vi "Data_analyzer_tester.vi"() -> ()   [LabVIEW 2021]
uses:
  <vilib>/DAQmx/create/channels.llb/DAQmx Create Channel (AI-Voltage-Basic).vi
  <vilib>/DAQmx/configure/timing.llb/DAQmx Timing (Sample Clock).vi
  <vilib>/daqmxs/DAQmx Read sim (Analog Wfm 1Chan NSamp).vi
  <vilib>/Waveform/WDTOps.llb/WDT Append Waveforms DBL.vi
  <vilib>/daqmxs/DAQmx sim.lvlib
panel:
  out "Prubeh frekvence":waveform(dbl)(graph)
  out "Pocet period":i32
  in  "Hystereze":dbl min=0.0 step=0.1
  in  "Uroven mereni":dbl
  in  "stop 2":bool
  out "Data":waveform(dbl)(graph)
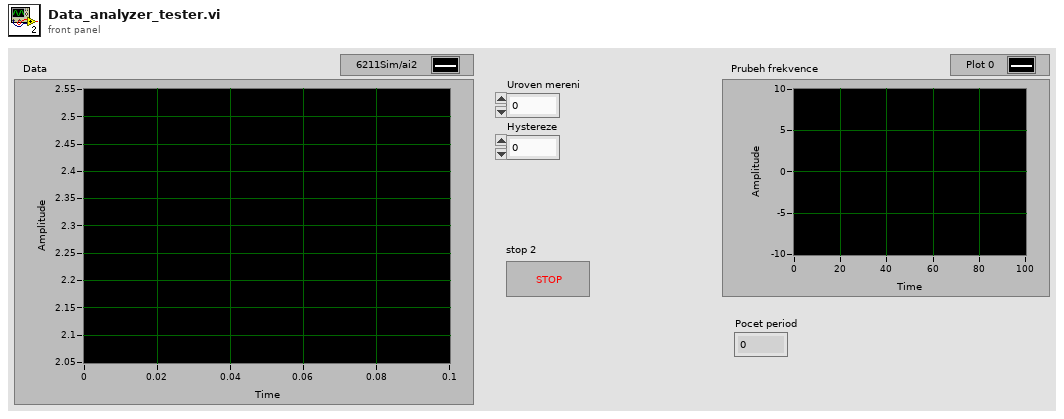
[diagram p1: front panel]
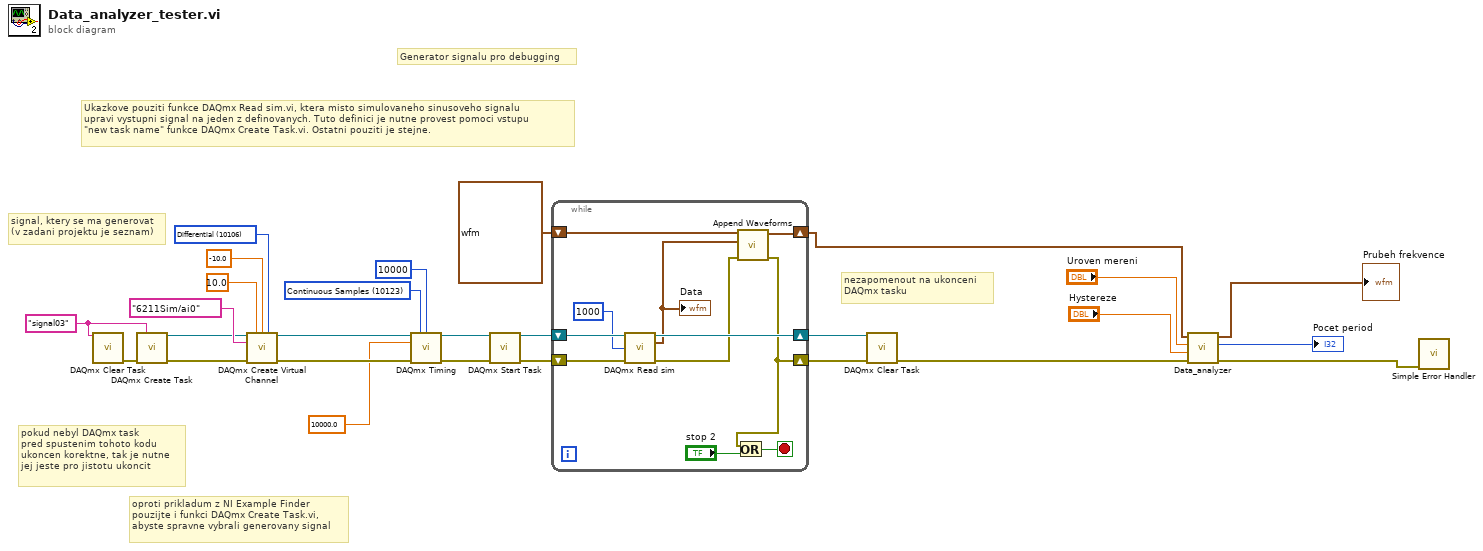
[diagram p0: block diagram]
diagram:
  w9 = "signal03"
  w15 = 10123 items=["Finite Samples"=10178, "Continuous Samples"=10123, "Hardware Timed Single Point"=12522] ("sample mode")
  w16 = 10106 items=["Default"=-1, "RSE"=10083, "NRSE"=10078, "Differential"=10106, "Pseudodifferential"=12529] ("input terminal configuration")
  # "nezapomenout na ukonceni\nDAQmx tasku"
  # "Ukazkove pouziti funkce DAQmx Read sim.vi, ktera misto simulovaneho sinusoveho signalu\nupravi vystupni signal na jeden z definovanych. Tuto definici je nutne provest pomoci vstupu\n\"new task name\" funkce DAQmx Create Task.vi. Ostatni pouziti je stejne."
  # "pokud nebyl DAQmx task\npred spustenim tohoto kodu\nukoncen korektne, tak je nutne\njej jeste pro jistotu ukoncit"
  # "signal, ktery se ma generovat\n(v zadani projektu je seznam)"
  # "oproti prikladum z NI Example Finder\npouzijte i funkci DAQmx Create Task.vi,\nabyste spravne vybrali generovany signal"
  # "Generator signalu pro debugging"
  n1 = call <vilib>:"DAQmx Clear Task.vi"("task in"=w9) -> ("error out"=w10:errorcluster)  [unwired: 14 in]
  n2 = call <vilib>:"DAQmx Create Task.vi"("new task name"=w9, "error in"=w10) -> ("task out"=w12:refnum<k21>, "error out"=w11:errorcluster)  [unwired: 12 in]
  n3 = call-poly <vilib>:"DAQmx Create Virtual Channel.vi"("task in"=w12, "maximum value"=10.0, "minimum value"=-10.0, "input terminal configuration"=w16, "physical channels"=tag "6211Sim/ai0", "error in"=w11) -> ("task out"=w27:refnum<k21>, "error out"=w26:errorcluster)  [unwired: 8 in]
  n4 = call-poly <vilib>:"DAQmx Timing.vi"("task/channels in"=w27, "sample mode"=w15, "samples per channel"=10000, "rate"=10000.0, "error in"=w26) -> ("task out"=w25:refnum<k21>, "error out"=w24:errorcluster)  [unwired: 9 in]
  n5 = call <vilib>:"DAQmx Start Task.vi"("task/channels in"=w25, "error in"=w24) -> ("task out"=w23:refnum<k21>, "error out"=w22:errorcluster)  [unwired: 12 in]
  n6 = while {
    shift-right: [w36] -> w20
    shift-left: w23 -> [w38]
    shift-right: [w30] -> w19
    shift-left: w22 -> [w37]
    shift-right: [w31] -> w2
    shift-left: waveform(dbl) {"t0"=timestamp(0 s since 1904-01-01), "dt"=1.0, "Y"=[]} ("waveform out") -> [w32]
    stop <- w33 stop-if-true
    n7 = call-poly <vilib>:"DAQmx Read sim.vi"("task/channels in"=w38, "number of samples per channel"=1000, "error in"=w37) -> ("task out"=w36:refnum<k21>, "data"=w28:waveform(dbl), "error out"=w29:errorcluster)  [unwired: 10 in]
    "Data" <- w28
    n8 = call-poly <vilib>:"Append Waveforms.vi"("error in (no error)"=w29, "waveform B"=w28, "waveform A"=w32) -> ("error out"=w30:errorcluster, "waveform out"=w31:waveform(dbl))  [unwired: 7 in]
    n9 = Or(x=w30, y="stop 2") -> (x .or. y?=w33:bool)
  }
  n10 = call <vilib>:"DAQmx Clear Task.vi"("task in"=w20, "error in"=w19) -> ("error out"=w8:errorcluster)  [unwired: 13 in]
  n11 = call "Data_analyzer.vi"("error in"=w8, "Hystereze"="Hystereze", "Uroven mereni"="Uroven mereni", "Data"=w2) -> ("error out"=w1:errorcluster, "Pocet period"=→"Pocet period":i32, "Prubeh frekvence"=→"Prubeh frekvence":waveform(dbl))  [unwired: 5 in]
  n12 = call <vilib>:"Simple Error Handler.vi"("error in (no error)"=w1) -> ()  [unwired: 4 in, 5 out]
